vi "Teleop Drivetrain Control.vi"(8 "Manip Button Cluster":T1, 9 "D-Pad":T2, 10 "Driver Button Cluster":T1, 11 "Axes":T3) -> ()   [LabVIEW 2015]
uses:
  Common Code/Gamepads/Axes Cluster.ctl
  Common Code/Gamepads/Button Cluster.ctl
  Common Code/Gamepads/D-Pad.ctl
  Common Code/Shot Type.ctl
  Common Code/Drivetrain Modes.ctl
  Common Code/Change Detect Boolean.vi
  Robot Global Data.vi
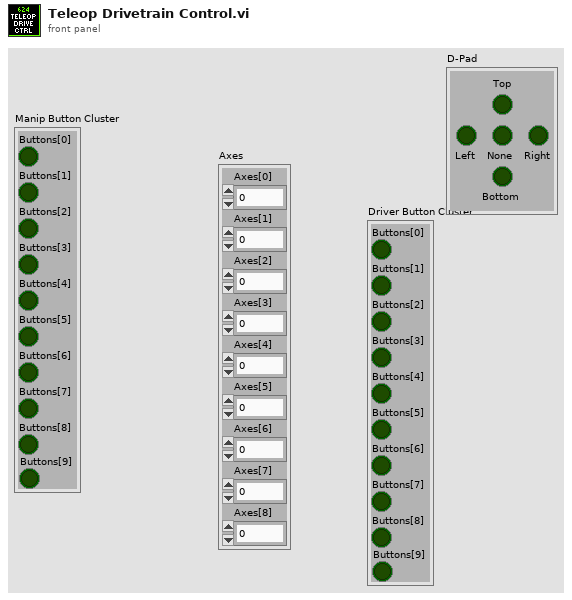
[diagram p1: front panel]
types:
  T1 = typedef "Button Cluster.ctl" = cluster{"Buttons[0]":bool, "Buttons[1]":bool, "Buttons[2]":bool, "Buttons[3]":bool, "Buttons[4]":bool, "Buttons[5]":bool, "Buttons[6]":bool, "Buttons[7]":bool, "Buttons[8]":bool, "Buttons[9]":bool}
  T2 = typedef "D-Pad.ctl" = cluster{"Top":bool, "Bottom":bool, "None":bool, "Right":bool, "Left":bool}
  T3 = typedef "Axes Cluster.ctl" = cluster{"Axes[0]":dbl, "Axes[1]":dbl, "Axes[2]":dbl, "Axes[3]":dbl, "Axes[4]":dbl, "Axes[5]":dbl, "Axes[6]":dbl, "Axes[7]":dbl, "Axes[8]":dbl}
  T4 = typedef "Drivetrain Modes.ctl" = enum16{"Tank", "Climb", "Manual", "Goal Vision Targeting", "PID Distance Drive", "Hybrid", "Gyro Steer"}
  T5 = typedef "Shot Type.ctl" = enum16{"Batter Shot", "Corner Shot", "Cleat Shot", "Vision Shot", "Deep Middle Shot"}
  T6 = typedef "Drivetrain Commands.ctl" = cluster{"Y Power":dbl, "Turn Power":dbl, "2nd Gear?":bool, "Modes":T4, "Heading Target":dbl, "X Max Speed":dbl, "Y Max Speed":dbl, "X Min Speed":dbl, "Y Min Speed":dbl, "Y Target":dbl, "Max Accel":dbl, "Max Velocity":dbl, "Y Power 2":dbl, "Pivot Speed":dbl}
  T7 = typedef "Shooter Command Cluster.ctl" = cluster{"Command":T8, "Mode":T9, "Shot Type":T5, "Override Trigger Sensor":bool, "Override Angle?":bool, "Hide From Death":bool}
  T8 = typedef "Shooter Commands.ctl" = enum16{"Idle", "Prime Shooter", "Shoot"}
  T9 = typedef "Shoot Modes Enum.ctl" = enum16{"Manual", "Safe", "Auto"}
  T10 = typedef "Climb Command Cluster.ctl" = cluster{"Climb Mode":T11, "Hold?":bool, "Manual State":T12}
  T11 = typedef "Climb Mode.ctl" = enum16{"Auto", "Semi-Auto", "Manual"}
  T12 = typedef "Climb Manual State.ctl" = cluster{"Release":bool, " PTO Engage":bool, "Extend":bool}
  T13 = typedef "Dashboard Control Data.ctl" = cluster{"Shooter Presets":T14, "Encoder Control":T16, "Steer PID output":cluster{"output high":dbl, "output low":dbl}, " Steer PID gains":cluster{"proportional gain (Kc)":dbl, "integral time (Ti, min)":dbl, "derivative time (Td, min)":dbl}, "Drivetrain Settings":T17, "Vision Packet":T18, "Dashboard Drivetrain Command":T19, "Info/Command Cluster":T21, "Ball Vision Packet":T22, "Intake Presets":T24, "Intake Encoder Control":T26, "Climb Presets":T27, "Goal Output Range":cluster{"output high":dbl, "output low":dbl}, "Enabled Systems":T28, "Auton Presets":T29, "Pressure M":dbl, "Pressure B":dbl, "Vision Timeout":dbl, "Auto-Shift":T30}
  T14 = typedef "Shooter Presets.ctl" = cluster{"Batter Shot":T15, "Deep Middle":T15, "Manual Shot":T15, "Left Ticks Per Rotation":dbl, "Right Ticks Per Rotation":dbl, "Low Bar Shot":T15, "Shooter RPM Tolerance":dbl, "Trigger Power":dbl, "Fire from Load Delay":i32, "Max Angle":dbl, "Min Angle":dbl, "Angle PID gains":cluster{"P":dbl, "I":dbl, "D":dbl}, "Angle Output":cluster{"output high":dbl, "output low":dbl}, "Shooter Angle Tolerance":dbl, "Vision Shoot x^2":dbl, "Vision Shoot x":dbl, "Feed Forward Max Accel":dbl, "Feed Forward Kv":dbl, "Backwards Trigger":dbl, "Shot Finish Delay (ms)":dbl, "Angle Max Current":dbl, "Angle Current Trip Time":dbl, "Intake Angle":dbl, "Vision Shoot c":dbl, "Reset?":bool, "Button Release Delay":dbl, "Angle Pot x":dbl, "Angle Pot c":dbl, "Ignore Angle?":bool, "Max RPM":dbl, "Safty Frist Angle":dbl, "Intake Danger Height":dbl, "Angle Pot B":i32, "Angle Pot M":dbl, "FF Finish RPM":dbl, "RPM PID Right":cluster{"P":dbl, "I":dbl, "D":dbl, "FF":dbl}, "RPM PID Left":cluster{"P":dbl, "I":dbl, "D":dbl, "FF":dbl}, "Backwards RPM":dbl, "Vision RPM":dbl, "Run Wheels Backward Delay":u32, "Cleat Shot":T15, "Vision Far RPM":dbl, "Vision Far Distance":dbl, "Vision Far Angle":dbl}
  T15 = typedef "Shot Presets.ctl" = cluster{"L":dbl, "R":dbl, "A":dbl}
  T16 = typedef "Encoder Control.ctl" = cluster{"Right Tick Constant":dbl, "Left Tick Constant":dbl, "Reset?":bool, "Y Dist":cluster{"PID gains":cluster{"proportional gain (Kc)":dbl, "integral time (Ti, min)":dbl, "derivative time (Td, min)":dbl}}, "Y Stop Thresh":dbl, "Y Stop Speed":dbl}
  T17 = typedef "Drivetrain Settings.ctl" = cluster{"Gyro Tolerance":dbl, "Throttle Ramp (ms)":dbl, "Kv":dbl, "Ka":dbl, "Feed Forward P":dbl, "Feed Forward D":dbl, "Goal Vision PID gains":cluster{"proportional gain (Kc)":dbl, "integral time (Ti, min)":dbl, "derivative time (Td, min)":dbl}, "Goal Detection Window":dbl, "Creep Rate":dbl, "Vision Throttle Threshold":dbl, "Min Turn Output":dbl, "Left Batter Angle":dbl, "Right Batter Angle":dbl}
  T18 = typedef "Goal Vision Packet.ctl" = cluster{"Distance":dbl, "Center X":dbl, "Center Y":dbl, "Found Target?":bool, "Robot Center":dbl, "Angle":dbl}
  T19 = typedef "Dashboard Drivetrain Command.ctl" = cluster{"Drivetrain Vision":T20}
  T20 = typedef "Drivetrain Vision.ctl" = cluster{"Goal Window":dbl, "Ball Window":dbl}
  T21 = typedef "Ball Tracking Command Cluster.ctl" = cluster{"Distance to Ball":dbl, "Desired Angle":dbl, "Command":enum16{"Turn to Ball", "Turn to Angle", "Get Distance"}, "Pixels from Center":dbl}
  T22 = typedef "Ball Vision Packet.ctl" = cluster{"Ball Detected?":bool, "Distance to Ball":dbl, "Desired Angle":dbl, "Pixels from Center":dbl, "Tracking mode":T23}
  T23 = typedef "Tracking Mode.ctl" = enum16{"Turn to Ball", "Turn to Angle"}
  T24 = typedef "Intake Presets.ctl" = cluster{"Intake Speed":dbl, "Outake Speed":dbl, "Low Height":dbl, "Half Height":dbl, "High Idle Height":dbl, "Angle Speed":dbl, "Angle Tolerance":dbl, "Encoder Scale":dbl, "Load Height":dbl, "Output Range":T25, "Rotation Power Max/Min":dbl, "MaxCurrent":dbl, "Intake Trip Time":dbl, "Idle Height":dbl, "Max Height":dbl, "Reset Encoders?":bool, "PID gains":cluster{"proportional gain (Kc)":dbl, "integral time (Ti, min)":dbl, "derivative time (Td, min)":dbl}, "Intake Stop Delay":u32, "Settle Time":dbl, "Settle Wait Time":dbl, "Pull Up Delay":dbl}
  T25 = typedef "Drivetrain Output Range.ctl" = cluster{"output high":dbl, "output low":dbl}
  T26 = typedef "IntakeEcoderControl.ctl" = cluster{"Arm Tick Constant":dbl, "Reset?":bool, "Y Dist":cluster{"PID gains":cluster{"proportional gain (Kc)":dbl, "integral time (Ti, min)":dbl, "derivative time (Td, min)":dbl}}, "Y Stop Thresh":dbl, "Y Stop Speed":dbl}
  T27 = typedef "Climb Presets.ctl" = cluster{"Pull Power":dbl, "Extend Power":dbl}
  T28 = typedef "Enabled Systems.ctl" = cluster{"Shoot":bool, "Intake":bool, "DT":bool, "Gyro":bool, "100ms":bool, "US":bool}
  T29 = typedef "Autonomous Presets.ctl" = cluster{"Pitch Limit":dbl, "Roll Limit":dbl, "Start Position":dbl, "Cross Position":dbl}
  T30 = typedef "Auto Shift Cluster.ctl" = cluster{"Delay":dbl, "Speed Thresh":dbl, "Upshift Accel":dbl, "Upshift Throttle":dbl, "Upshift Throttle Accel":dbl, "Downshift Throttle":dbl, "Downshift Throttle Accel":dbl, "Pressure Threshold":dbl}
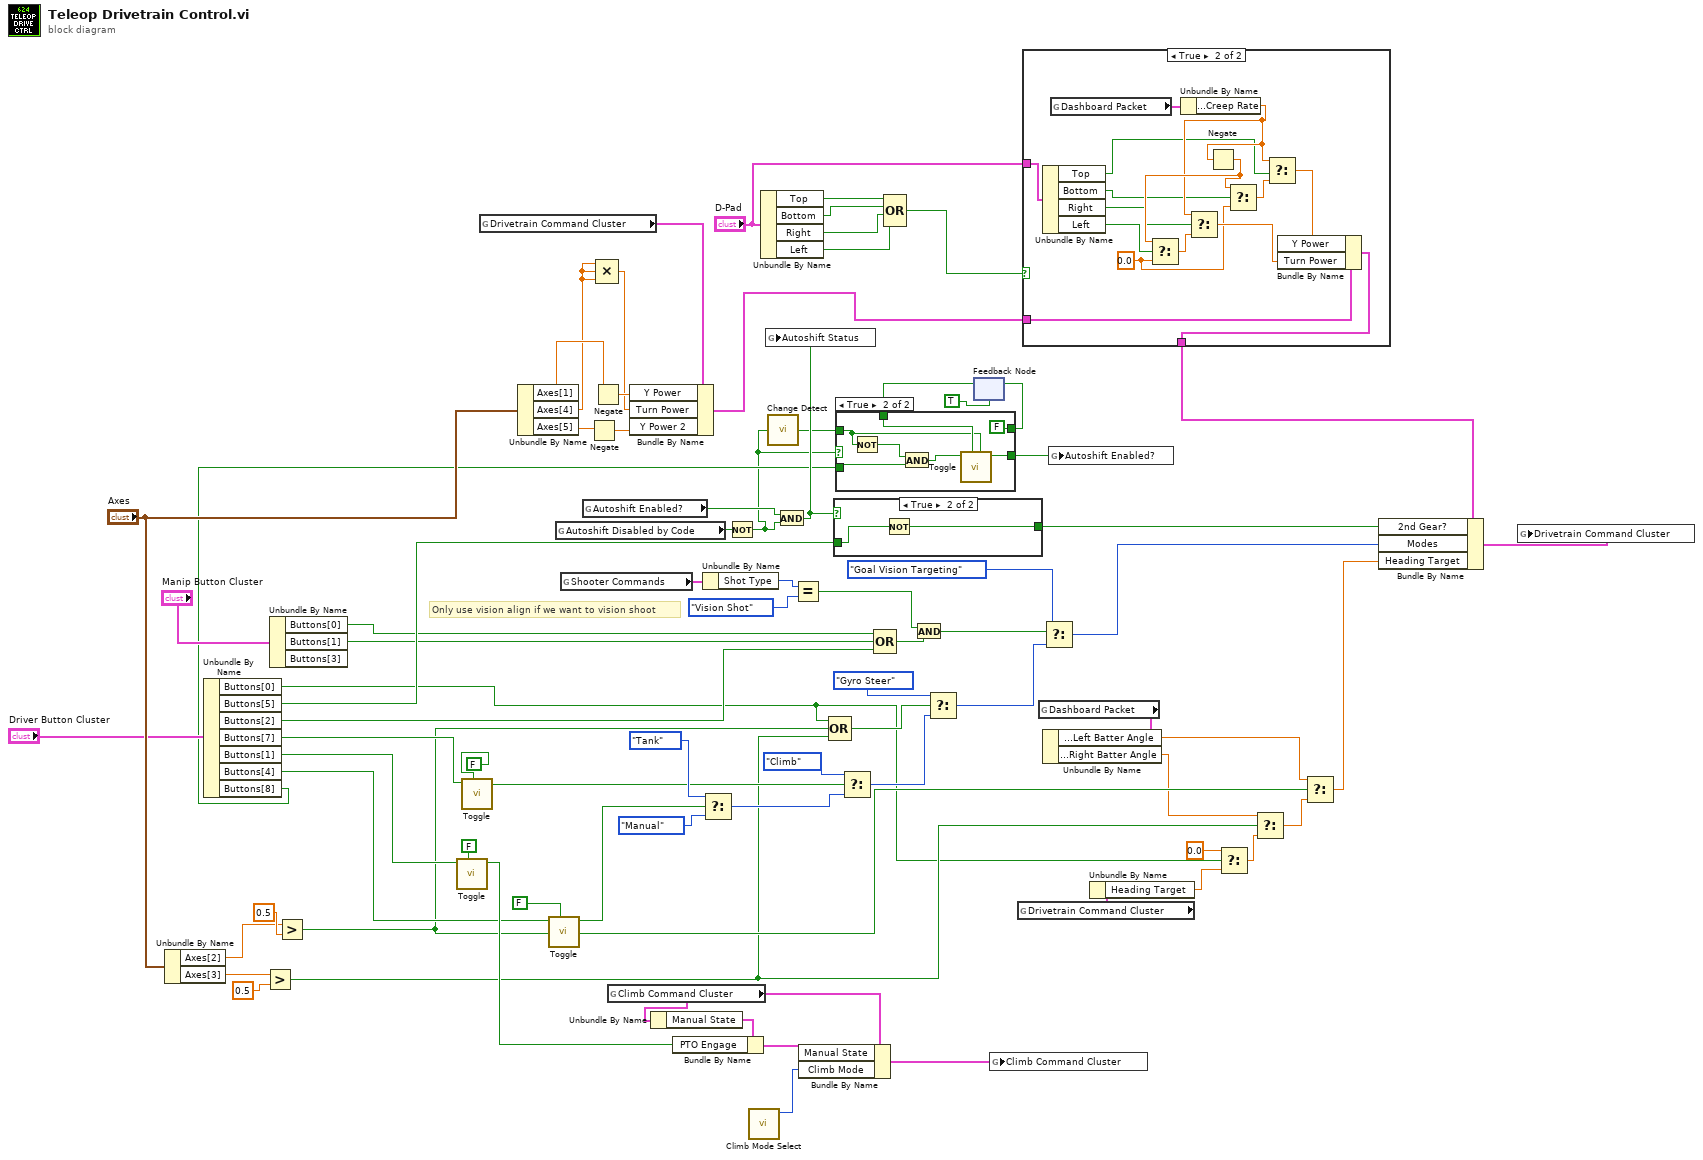
[diagram p0: block diagram]
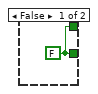
[diagram p2: hidden frame]
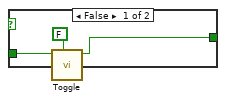
[diagram p3: hidden frame]
diagram:
  # "Only use vision align if we want to vision shoot"
  n1 = Unbundle By Name("Axes") -> ("Axes[2]"=w37:dbl, "Axes[3]"=w51:dbl)
  n2 = Unbundle By Name("Driver Button Cluster") -> ("Buttons[0]"=w16:bool, "Buttons[5]"=w74:bool, "Buttons[2]"=w57:bool, "Buttons[7]"=w53:bool, "Buttons[1]"=w73:bool, "Buttons[4]"=w20:bool, "Buttons[8]"=w7:bool)
  n3 = Greater?(x=w51, y=0.5) -> (0:w18:bool)
  n4 = Unbundle By Name("Manip Button Cluster") -> ("Buttons[0]"=w58:bool, "Buttons[1]"=w62:bool)  [unwired: 1 out]
  n5 = Greater?(x=w37, y=0.5) -> (0:w19:bool)
  n6 = call "Toggle.vi"("Initial Value"=FALSE, "In"=w73) -> ("Toggled"=w68:bool)  [unwired: 9 in]
  n7 = call "Toggle.vi"("Initial Value"=FALSE, "In"=w53) -> ("Toggled"=w30:bool)  [unwired: 9 in]
  n8 = global read "Robot Global Data.vi" "Drivetrain Command Cluster"() -> (w33:T6)
  n9 = Unbundle By Name("Axes") -> ("Axes[1]"=w34:dbl, "Axes[4]"=w29:dbl, "Axes[5]"=w32:dbl)
  n10 = call "Toggle.vi"("Initial Value"=FALSE, "In"=w20) -> ("Toggled"=w36:bool)  [unwired: 9 in]
  n11 = global read "Robot Global Data.vi" "Autoshift Disabled by Code"() -> (w10:bool)
  n12 = global read "Robot Global Data.vi" "Shooter Commands"() -> (w78:T7)
  n13 = global read "Robot Global Data.vi" "Autoshift Enabled?"() -> (w9:bool)
  n14 = Negate(x=w32) -> (-x=w31:dbl)
  n15 = Negate(x=w34) -> (-x=w35:dbl)
  n16 = Compound Arithmetic op=MULTIPLY(w29, w29, w29) -> (w28:dbl)
  n17 = global read "Robot Global Data.vi" "Climb Command Cluster"() -> (w46:T10)
  n18 = Bundle By Name(cluster=w33, "Y Power"=w35, "Turn Power"=w28, "Y Power 2"=w31) -> (w44:T6)
  n19 = Unbundle By Name(w46) -> ("Manual State"=w67:T12)
  n20 = Bundle By Name(cluster=w67, "PTO Engage"=w68) -> (w48:T12)
  n21 = Unbundle By Name(w78) -> ("Shot Type"=w77:T5)
  n22 = Select(t=Drivetrain_Modes."Tank", s=w36, f=Drivetrain_Modes."Manual" ("Modes")) -> (s? t:f=w55:T4)
  n23 = Not(x=w10) -> (.not. x?=w5:bool)
  n24 = call "Climb Mode Select.vi"() -> ("Mode"=w47:T11)  [unwired: 11 in]
  n25 = Unbundle By Name("D-Pad") -> ("Top"=w43:bool, "Bottom"=w42:bool, "Right"=w41:bool, "Left"=w40:bool)
  n26 = call-poly "Change Detect.vi"("In"=w5) -> ("Changed?"=w4:bool)
  n27 = And(x=w9, y=w5) -> (x .and. y?=w8:bool)
  n28 = global write "Robot Global Data.vi" "Autoshift Status"(w8) -> ()
  n29 = Equal?(x=w77, y=Shot_Type."Vision Shot") -> (x = y?=w59:bool)
  n30 = Bundle By Name(cluster=w46, "Manual State"=w48, "Climb Mode"=w47) -> (w49:T10)
  n31 = Compound Arithmetic op=OR(w16, w19, w18) -> (w21:bool)
  n32 = case shown="True" w8 {
    tunnel: [w83 w85] -> w80
    tunnel: w74 -> [w82 w84]
    frame False {
      n33 = call "Toggle.vi"("Initial Value"=FALSE, "In"=w82) -> ("Toggled"=w83:bool)  [unwired: 9 in]
    }
    frame True {
      n34 = Not(x=w84) -> (.not. x?=w85:bool)
    }
  }
  n35 = Select(t=Drivetrain_Modes."Climb" ("s? t:f"), s=w30, f=w55) -> (s? t:f=w27:T4)
  n36 = Compound Arithmetic op=OR(w58, w62, w57) -> (w63:bool)
  n37 = Compound Arithmetic op=OR(w43, w42, w41, w40) -> (w38:bool)
  n38 = And(x=w59, y=w63) -> (x .and. y?=w61:bool)
  n39 = Select(t=Drivetrain_Modes."Gyro Steer", s=w21, f=w27) -> (s? t:f=w26:T4)
  n40 = feedback #1(TRUE ("Initial Value")) -> (w2:bool)
  n41 = case shown="True" w5 {
    tunnel: w7 -> [_ w91]
    tunnel: [w86 w93] -> w6
    tunnel: w4 -> [_ w88]
    tunnel: w2 -> [_ w89]
    tunnel: [w86 FALSE ("Toggled")] -> w1
    frame False {
      w86 = FALSE ("Toggled")
    }
    frame True {
      n42 = Not(x=w88) -> (.not. x?=w92:bool)
      n43 = And(x=w92, y=w91) -> (x .and. y?=w90:bool)
      n44 = call "Toggle.vi"("Reinit?"=w88, "Initial Value"=w89, "In"=w90) -> ("Toggled"=w93:bool)  [unwired: 8 in]
    }
  }
  n45 = feedback-in #1(w1) -> ()
  n46 = global write "Robot Global Data.vi" "Climb Command Cluster"(w49) -> ()
  n47 = global read "Robot Global Data.vi" "Drivetrain Command Cluster"() -> (w23:T6)
  n48 = case shown="True" w38 {
    tunnel: w44 -> [w94 w108]
    tunnel: [w94 w109] -> w45
    tunnel: "D-Pad" -> [_ w96]
    frame False {
    }
    frame True {
      w95 = 0.0 ("f")
      n49 = Unbundle By Name(w96) -> ("Top"=w100:bool, "Bottom"=w99:bool, "Right"=w98:bool, "Left"=w97:bool)
      n50 = global read "Robot Global Data.vi" "Dashboard Packet"() -> (w103:T13)
      n51 = Unbundle By Name(w103) -> ("Drivetrain Settings.Creep Rate"=w104:dbl)
      n52 = Negate(x=w104) -> (-x=w105:dbl)
      n53 = Select(t=w105, s=w97, f=w95) -> (s? t:f=w101:dbl)
      n54 = Select(t=w104, s=w98, f=w101) -> (s? t:f=w102:dbl)
      n55 = Select(t=w105, s=w99, f=w95) -> (s? t:f=w106:dbl)
      n56 = Select(t=w104, s=w100, f=w106) -> (s? t:f=w107:dbl)
      n57 = Bundle By Name(cluster=w108, "Y Power"=w107, "Turn Power"=w102) -> (w109:T6)
    }
  }
  n58 = global read "Robot Global Data.vi" "Dashboard Packet"() -> (w24:T13)
  n59 = Unbundle By Name(w24) -> ("Drivetrain Settings.Left Batter Angle"=w22:dbl, "Drivetrain Settings.Right Batter Angle"=w13:dbl)
  n60 = Select(t=Drivetrain_Modes."Goal Vision Targeting", s=w61, f=w26) -> (s? t:f=w56:T4)
  n61 = global write "Robot Global Data.vi" "Autoshift Enabled?"(w6) -> ()
  n62 = Unbundle By Name(w23) -> ("Heading Target"=w15:dbl)
  n63 = Select(t=0.0, s=w16, f=w15) -> (s? t:f=w14:dbl)
  n64 = Select(t=w13, s=w18, f=w14) -> (s? t:f=w17:dbl)
  n65 = Select(t=w22, s=w19, f=w17) -> (s? t:f=w11:dbl)
  n66 = Bundle By Name(cluster=w45, "2nd Gear?"=w80, "Modes"=w56, "Heading Target"=w11) -> (w79:T6)
  n67 = global write "Robot Global Data.vi" "Drivetrain Command Cluster"(w79) -> ()
